vi "CRYLegend Resize in Graph Window.vi"(8 "VScrollShow":bool=TRUE, 9 "Pane Ref":refnum<vi>, 10 "input cluster":T1, 11 "Legend":refnum<vi>) -> ()   [LabVIEW 2013]
uses:
  <vilib>/Utility/miscctls.llb/LVRectTypeDef.ctl
  <vilib>/Utility/miscctls.llb/LVBoundsTypeDef.ctl
  <vilib>/Utility/miscctls.llb/LVRowAndColumnTypeDef.ctl
  <vilib>/Utility/miscctls.llb/LVPositionTypeDef.ctl
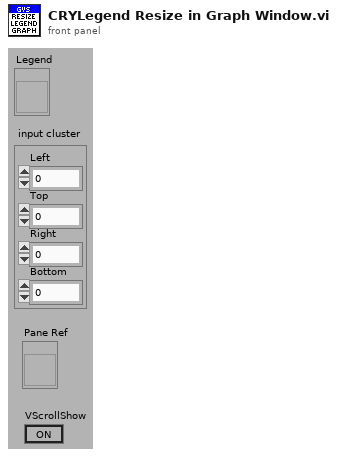
[diagram p1: front panel]
types:
  T1 = typedef "LVRectTypeDef.ctl" = cluster{"Left":i16, "Top":i16, "Right":i16, "Bottom":i16}
  T2 = typedef "LVPointTypeDef.ctl" = cluster{"Horizontal":i16, "Vertical":i16}
  T3 = typedef "LVRowAndColumnTypeDef.ctl" = cluster{"Row":i32, "Column":i32}
  T4 = typedef "LVBoundsTypeDef.ctl" = cluster{"Width":u32, "Height":u32}
  T5 = typedef "LVPositionTypeDef.ctl" = cluster{"Left":i32, "Top":i32}
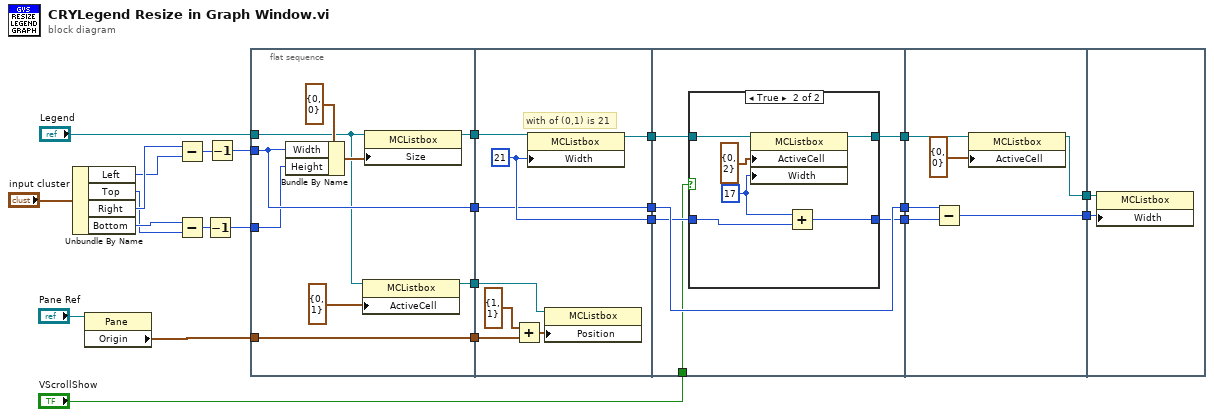
[diagram p0: block diagram]
diagram:
  n1 = Unbundle By Name("input cluster") -> ("Left"=w16:i16, "Top"=w15:i16, "Right"=w22:i16, "Bottom"=w21:i16)
  n2 = property class="Pane"(reference="Pane Ref") -> ("Origin"=w8:T2)  [unwired: 1 in, 2 out]
  n3 = Subtract(x=w22, y=w16) -> (x-y=w19:i16)
  n4 = Subtract(x=w21, y=w15) -> (x-y=w20:i16)
  n5 = Decrement(x=w20) -> (x-1=w18:i16)
  n6 = Decrement(x=w19) -> (x-1=w17:i16)
  n7 = flat-sequence {
    tunnel: w18 -> [w31]
    tunnel: w17 -> [w32]
    tunnel: [w32] -> w25
    tunnel: w8 -> [w30]
    tunnel: [w30] -> w24
    tunnel: "Legend" -> [w27]
    tunnel: [w28] -> w12
    tunnel: [w26] -> w10
    tunnel: w25 -> [w38]
    tunnel: w24 -> [w41]
    tunnel: [w38] -> w7
    tunnel: [w39] -> w5
    tunnel: w12 -> [w37]
    tunnel: [w36] -> w3
    tunnel: w10 -> [w35]
    tunnel: w7 -> [w46]
    tunnel: [w46] -> w6
    tunnel: w5 -> [w45]
    tunnel: [w44] -> w4
    tunnel: w3 -> [w48]
    tunnel: [w47] -> w2
    tunnel: "VScrollShow" -> [w43]
    tunnel: w6 -> [w61]
    tunnel: w4 -> [w60]
    tunnel: [w57] -> w23
    tunnel: w2 -> [w59]
    tunnel: [w58] -> w11
    tunnel: w23 -> [w64]
    tunnel: w11 -> [w63]
    frame #0 {
      n8 = Bundle By Name(cluster=T4 {"Width"=0, "Height"=0} ("Size"), "Width"=w32, "Height"=w31) -> (w33:T4)
      n9 = property on="Property Node" class="MCListbox"(reference=w27, "ActiveCell"=T3 {"Row"=0, "Column"=1} ("Active Cell:Active Cell")) -> (reference out=w26:refnum<vi>)  [unwired: 1 in, 1 out]
      n10 = property on="Property Node" class="MCListbox"(reference=w27, "Size"=w33) -> (reference out=w28:refnum<vi>)  [unwired: 1 in, 1 out]
    }
    frame #1 {
      w39 = u32 21 ("Active Cell:Cell Size:Width")
      # "with of (0,1) is 21"
      n11 = Add(x=T5 {"Left"=1, "Top"=1} ("Position"), y=w41) -> (x+y=w42:T5)
      n12 = property on="Property Node" class="MCListbox"(reference=w37, "Width"=w39) -> (reference out=w36:refnum<vi>)  [unwired: 1 in, 1 out]
      n13 = property on="Property Node" class="MCListbox"(reference=w35, "Position"=w42) -> ()  [unwired: 1 in, 2 out]
    }
    frame #2 {
      n14 = case shown="True" w43 {
        tunnel: w48 -> [w50 w56]
        tunnel: [w50 w55] -> w47
        tunnel: w45 -> [w49 w52]
        tunnel: [w49 w51] -> w44
        frame False {
        }
        frame True {
          w53 = u32 17 ("Active Cell:Cell Size:Width")
          n15 = property on="Property Node" class="MCListbox"(reference=w56, "ActiveCell"=T3 {"Row"=0, "Column"=2} ("Active Cell:Active Cell"), "Width"=w53) -> (reference out=w55:refnum<vi>)  [unwired: 1 in, 1 out]
          n16 = Add(x=w53, y=w52) -> (x+y=w51:u32)
        }
      }
    }
    frame #3 {
      n17 = Subtract(x=w61, y=w60) -> (x-y=w57:u32)
      n18 = property on="Property Node" class="MCListbox"(reference=w59, "ActiveCell"=T3 {"Row"=0, "Column"=0} ("Active Cell:Active Cell")) -> (reference out=w58:refnum<vi>)  [unwired: 1 in, 1 out]
    }
    frame #4 {
      n19 = property on="Property Node" class="MCListbox"(reference=w63, "Width"=w64) -> ()  [unwired: 1 in, 2 out]
    }
  }
